vi "TypesetInsideMathmode.vi"(11 "X Axis Name":string) -> (2 "Mathmode String":string, 3 "De-dollared String":string)   [LabVIEW 2012]
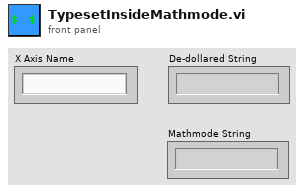
[diagram p1: front panel]
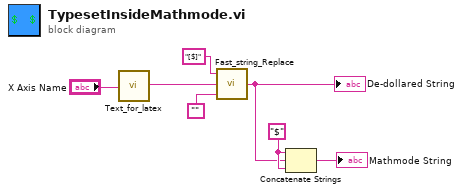
[diagram p0: block diagram]
diagram:
  w3 = "$" ("string")
  n1 = call "Text_for_latex.vi"("Input String"="X Axis Name") -> ("Output String"=w4:string)
  n2 = call "Fast_string_Replace.vi"("Replace match with:"="", "Input String"=w4, "regular expression"="[$]") -> ("Output String"=w2:string)  [unwired: 2 out]
  "De-dollared String" <- w2
  n3 = Concatenate Strings(w3, w2, w3) -> (→"Mathmode String":string)
